vi "Tabla Productos.vi"(0 "stop":bool, 9 "Multicolumn Listbox":i32(listbox), 10 "Producto_precio_inventario":string[][](array[string])=[["Confleis", "$50", "15"], ["Compemiso", "$1", "15"], ["Saludo", "$10.5", "100"]]) -> (2 "Product selection 2":string[](array[string]))   [LabVIEW 2019, in "Products.lvlib"]
uses:
  Products.lvlib
panel:
  in  "Multicolumn Listbox 2":i32(listbox)
  out "Product selection":string[](array[string])
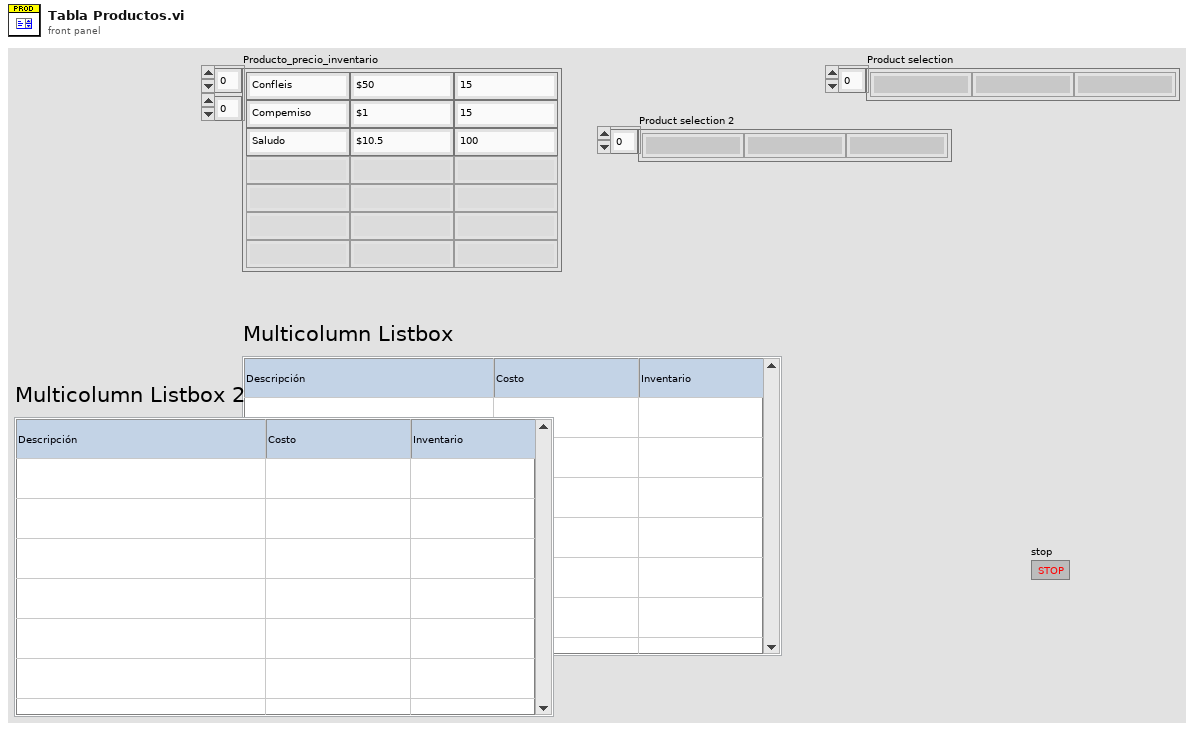
[diagram p1: front panel]
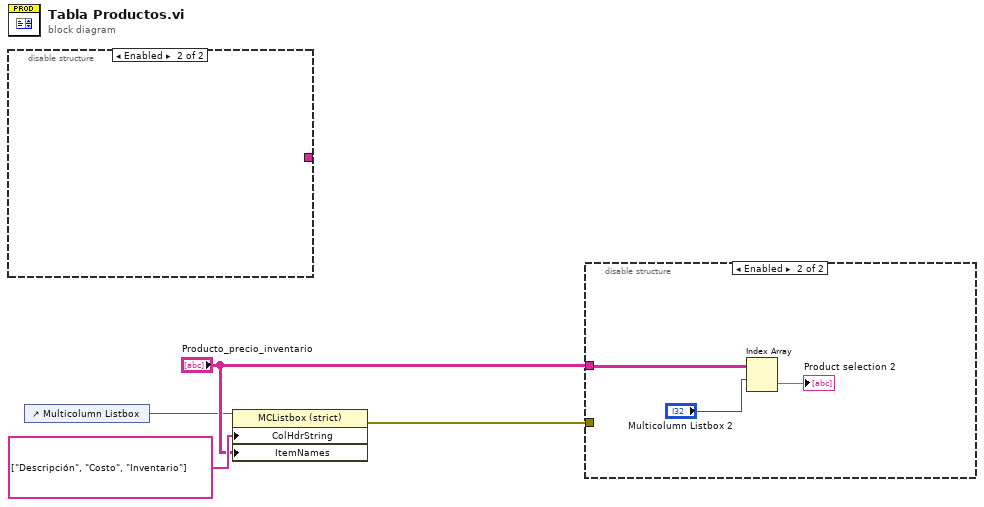
[diagram p0: block diagram]
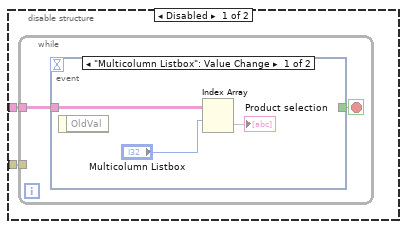
[diagram p2: hidden frame]
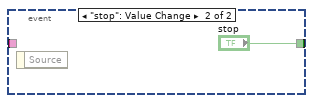
[diagram p3: hidden frame]
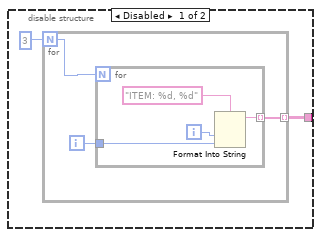
[diagram p4: hidden frame]
diagram:
  n1 = disable-structure shown="Enabled" {
    disable-tunnel: [w5 _] -> _
    frame Disabled {
      n2 = for {
        N: 3 -> [w9]
        tunnel: [w8] -> w5 mode=indexing
        i -> [w7]
        n3 = for {
          N: w9 -> [_]
          tunnel: [w12] -> w8 mode=indexing
          tunnel: w7 -> [w11]
          i -> [w13]
          n4 = Format Into String(format string="ITEM: %d, %d", w13, w11) -> (resulting string=w12:string)  [unwired: 2 in, 1 out]
        }
      }
    }
    frame Enabled {
    }
  }
  n5 = control-ref of="Multicolumn Listbox"() -> (w1:refnum<vi>)
  n6 = property class="MCListbox (strict)"(reference=w1, "ColHdrString"=string[] ["Descripción", "Costo", "Inventario"] ("Column Header Strings[]"), "ItemNames"="Producto_precio_inventario") -> (error out=w3:errorcluster)  [unwired: 1 in, 1 out]
  n7 = disable-structure shown="Enabled" {
    disable-tunnel: w3 -> [w15 _]
    disable-tunnel: "Producto_precio_inventario" -> [w14 w22]
    frame Disabled {
      n8 = while {
        tunnel: w15 -> [_]
        tunnel: w14 -> [w17]
        stop <- w16 stop-if-true
        n9 = event shown="[0] \"Multicolumn Listbox\": Value Change" {
          selector: _ -> [_ _]
          dyn-events: _ -> [_ _]
          timeout: _ -> [_ _]
          tunnel: w17 -> [w20 _]
          tunnel: [_ "stop"] -> w16
          event "Multicolumn Listbox": Value Change {
            n10 = event-data() -> ()  [unwired: 1 in, 1 out]
            n11 = Index Array(array=w20, index (row)="Multicolumn Listbox") -> (element=→"Product selection":string[])  [unwired: 1 in]
          }
          event "stop": Value Change {
            n12 = event-data() -> ()  [unwired: 1 in, 1 out]
          }
        }
      }
    }
    frame Enabled {
      n13 = Index Array(array=w22, index (row)="Multicolumn Listbox 2") -> (element=→"Product selection 2":string[])  [unwired: 1 in]
    }
  }
